vi "Close.vi"(8 "error in (no error)":errorcluster, 11 "Data in":refnum<class "conc_SharedVar_I8.lvclass">) -> (0 "error out":errorcluster, 3 "Data out":refnum<class "conc_SharedVar_I8.lvclass">)   [LabVIEW 2021, in "conc_SharedVar_I8.lvclass"]
uses:
  conc_SharedVar_I8.lvclass
  conc_SharedVar_I8.lvclass/conc_SharedVar_I8.ctl
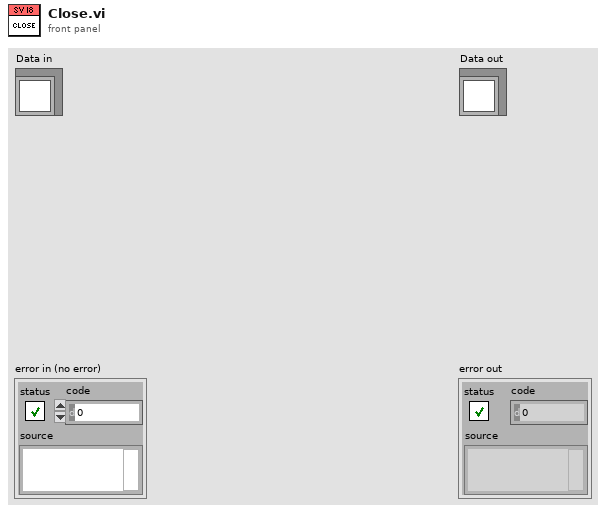
[diagram p1: front panel]
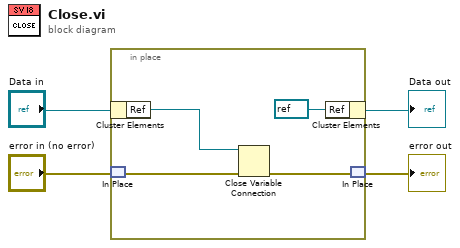
[diagram p0: block diagram]
diagram:
  n1 = in-place {
    n2 = in-place-cluster #1("Data in") -> ("Ref"=w8:refnum<k21>)
    n3 = in-place-match #2("error in (no error)") -> (w7:errorcluster)
    n4 = Close Variable Connection(8:w7, 11:w8) -> (0:w6:errorcluster)
    n5 = in-place-cluster #1("Ref"=refnum<k21> refnum) -> (→"Data out":refnum<class "conc_SharedVar_I8.lvclass">)
    n6 = in-place-match #2(w6) -> (→"error out":errorcluster)
  }
